vi "AlliGator Select FLI Channel Type.vi"(0 "Available Channel Names":string[](array[string]), 11 "error in (no error)":errorcluster) -> (1 "Dataset Channel":T1, 2 "Available Channel Names":string[](array[string]), 3 "Complementary Channel Name":string, 4 "Selected Channel Name":string, 6 "Channel Arithmetic":T2, 10 "G2 Channel Name (or single Gate Name)":string, 13 "Selected Channel Message":string, 14 "INT Channel Name (or empty)":string, 15 "error out":errorcluster)   [LabVIEW 2021, in "AlliGator Dual-Channel Datasets.lvlib"]
doc: "Used when loading a new dataset. If the selected channel name is compatible, use it, if not either open a dialog (dual-channel dataset) or use the default (single-channel dataset)."
uses:
  AlliGator Dual-Channel Datasets.lvlib
  AlliGator Gate Arithmetic.ctl
  AlliGator Dataset Channel.ctl
  AlliGator Settings List.ctl
  Variant/Variant to Data/Variant to [String].vi
  Variant/Variant to Data/Variant to U16.vi
  AlliGator Settings.lvlib
  Variant/Variant to Data/Variant to Data.lvlib
  AlliGator HDF5.lvlib
  AlliGator Files.lvlib
panel:
  out "Cancelled?":bool
  # "see the AlliGator License on the block diagram (Ctrl+E or Window:Show Block Diagram)"
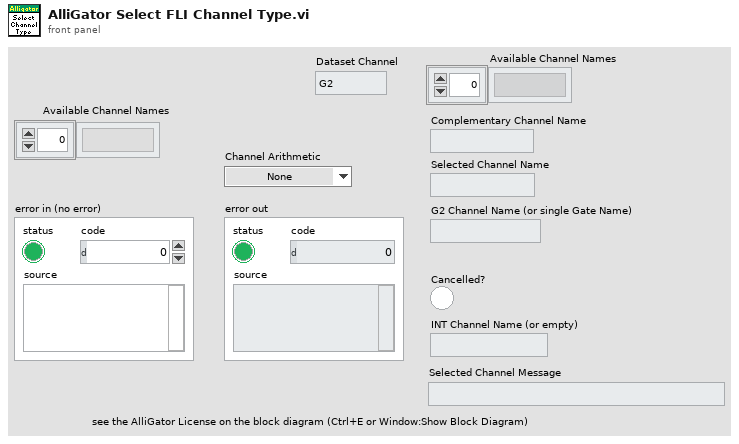
[diagram p1: front panel]
types:
  T1 = typedef "AlliGator Dual-Channel Datasets.lvlib/AlliGator Dataset Channel.ctl" = enum16{"G2", "INT"}
  T2 = typedef "AlliGator Settings.lvlib/AlliGator Gate Arithmetic.ctl" = enum16{"None", "INT-G2", "G2/INT*<INT>", "(1 - G2/INT)*<INT>"}
  T3 = typedef "AlliGator Settings.lvlib/AlliGator Settings List.ctl" = enum16{"GUI:Visible Settings Tab", "GUI:Last Run Version", "Source Image:Use Image Histogram for Contrast", "Source Image:Low Count Pixels Rejection Options", "Source Image:High Count Pixels Rejection Options", "Source Image:Use Image Brightness", "Source Image:Blend Overlay with Image Background", "Source Image:Use Fixed ROI Diameter", "Source Image:ROI Diameter", "Source Image:ROI Center Color", "Source Image:Peak Threshold", "Source Image:Intensity Threshold", "Source Image:Image Binning Options", "Source Image:Image Smoothing Options", "Source Image:Image Histogram Active", "Source Image:Invert Binary Mask", "Source Image:Hot Pixel Removal", "Source Image:Overlay Analyzed ROI Center", "Source Image:Auto-Adjust Contrast", "Source Image:Histogram Lower Percentile", "Source Image:Histogram Upper Percentile", "Source Image:Save Source Image", "Source Image:Scale Bar Options", "Source Image:Image Resolution (Pixel Size)", "Source Image:Flatfield Correction", "Source Image:Show Dead Left Columns Correction", "Source Image:Dead Left Columns Correction", "Source Image:Image Pre-Processing Operations Order", "Data Information:Gate Width", "Data Information:Nanotime Gate Separation", "Data Information:Macrotime Gate Separation", "Data Information:Gate Step", "Data Information:# Gates", "Data Information:Gate Image Exposure", "Data Information:Gate Image Integration", "Data Information:Gates to Skip", "Data Information:Gates to Keep", "Data Information:Define Gates to", "Data Information:Channel Name", "Data Information:Available Channel Names", "Data Information:Channel Arithmetic", "Data Information:Background File Subtraction", "Data Information:Background File", "Data Information:Background Scaling Factor", "Data Information:Background Pile-up Correction", "Data Information:Background Pixel Well Capacity", "Data Information:Laser Period", "Data Information:SYNC Period", "Data Information:Pile-up Correction", "Data Information:Pixel Well Capacity", "Data Information:Dataset Scaling Factor", "Fluorescence Decay_Decay Pre-Processing:Reverse Gates", "Fluorescence Decay_Decay Pre-Processing:Verbose Decay Pre-Processing", "Fluorescence Decay_Decay Pre-Processing:Use Decay Pre-Processing", "Fluorescence Decay_Decay Pre-Processing:Background Subtraction", "Fluorescence Decay_Decay Pre-Processing:Background Definition Range", "Fluorescence Decay_Decay Pre-Processing:Baseline Subtraction Method", "Fluorescence Decay_Decay Pre-Processing:Decay Pre-Processing Operations Order", "Fluorescence Decay_Decay Pre-Processing:Smoothing Parameter", "Fluorescence Decay_Decay Pre-Processing:Shift Decay", "Fluorescence Decay_Decay Pre-Processing:Decay Shift Parameters", "Fluorescence Decay_Decay Pre-Processing:Fold Decay", "Fluorescence Decay_Decay Pre-Processing:# Folds", "Fluorescence Decay_Decay Pre-Processing:1-Normalize Decay", "Fluorescence Decay_Decay Pre-Processing:[0-1]-Normalize Decay", "Fluorescence Decay_Decay Pre-Processing:Smoothen Decay", "Fluorescence Decay_Decay Pre-Processing:Extrapolate Decay", "Fluorescence Decay_Decay Pre-Processing:Use Periodicity", "Fluorescence Decay_Decay Pre-Processing:Use Cursors", "Fluorescence Decay_Decay Pre-Processing:Tail Fraction", "Fluorescence Decay_Decay Pre-Processing:Head Fraction", "Fluorescence Decay_Decay Pre-Processing:Additional Points", "Fluorescence Decay_Decay Pre-Processing:Straighten Decay", "Fluorescence Decay_Decay Pre-Processing:Constant Background", "Fluorescence Decay_Decay Pre-Processing:Pixel-Normalize Decay", "Fluorescence Decay_Advanced Analysis:Extract IRF instead of Decay", "Fluorescence Decay_Advanced Analysis:IRF Extraction Options", "Fluorescence Decay_Advanced Analysis:IRF Optimization Options", "Fluorescence Decay_Advanced Analysis:Square Pulse Options", "Fluorescence Decay_Advanced Analysis:IRF Order", "Fluorescence Decay_Advanced Analysis:IRF Time Constants", "Fluorescence Decay_Advanced Analysis:Wavelet Analysis Options", "Fluorescence Decay_Advanced Analysis:Average Lifetime Options", "Fluorescence Decay_Fit Options:Fit Options", "Fluorescence Decay_Fit Options:Use Legacy Fitting Approach", "Fluorescence Decay_Fit Options:Use Data Information Laser Period", "Fluorescence Decay_Fit Parameters:Displayed Fit Parameters", "Fluorescence Decay_Fit Parameters:Fit Parameter Constraints", "Fluorescence Decay_Fit Parameters:Export Tabulated Results", "Fluorescence Decay_Fit Parameters:MLE Baseline Offset Type", "Fluorescence Decay_Fit Parameters:MLE Baseline Offset", "Fluorescence Decay_Fit Parameters:Guess Parameter Names", "Fluorescence Decay_Fit Parameters:Guess Parameter Values", "Fluorescence Decay_Fit Parameters:Guess Parameters Options", "Fluorescence Decay_Styles:Show Last Decay Only", "Fluorescence Decay_Styles:Decay Graph Color Array", "Fluorescence Decay:Decay Graph Active", "Fluorescence Decay Statistics:Min Peak Value", "Fluorescence Decay Statistics:Reject Low Decay Peak Pixels", "Fluorescence Decay Statistics:Reject High Decay Peak Pixels", "Fluorescence Decay Statistics:Max Peak Value", "Time Traces:Use File Timestamp", "Time Traces:Time Step", "Time Traces:Use Intensity Correction File", "Time Traces:Intensity Correction File", "Phasor Plot:Phasor Plot Smoothing Options", "Phasor Plot:Phasor Plot Size", "Phasor Plot:Phasor Plot Graphics Options", "Phasor Plot:Cumulative Phasor Plot", "Phasor Plot:Use Phasor Brightness", "Phasor Plot:Blend Overlay with Phasor Background", "Phasor Plot:Save Phasor Plot", "Phasor Plot:Show References", "Phasor Plot:Phasor Ratio Decay Range", "Phasor Plot:Exponential Fading", "Phasor Plot:Phasor Ratio Reference Colors", "Phasor Plot:Reference Radius", "Phasor Plot:Show Color Map Vertices", "Phasor Plot:Phasor Plot Active", "Phasor Plot:Phasor Ratio Color Map Type", "Phasor Plot:Phasor Ratio Color Map", "Phasor Plot:Phasor Ratio Display Range", "Phasor Plot:Selected Image ROI(s)", "Phasor Plot:All Image ROIs", "Phasor Plot:Selected Phasor Plot ROI(s)", "Phasor Plot:All Phasor Plot ROIs", "Phasor Plot:Phasor Ratio Color-Coded Quantity", "Phasor Plot:Store Phasor Harmonics", "Phasor Plot:Draw Reference Segment", "Phasor Plot:User-Defined Quantity", "Phasor Graph:Phasor Frequency", "Phasor Graph:Phasor Ratio Type", "Phasor Graph:Pixel-level Phasor Computation", "Phasor Graph:Save Phasor Graph", "Phasor Graph:Phasor Graph Active", "Phasor Graph:Phasor SDV Options", "Phasor Calibration:Use Backup Calibration if needed", "Phasor Graph:Define Shortest Lifetime as", "Phasor Calibration:Backup Calibration Type", "Phasor Calibration:Calibration Type", "Phasor Calibration:Calibration Lifetime", "Phasor Calibration:Calibration Map Algorithm", "Single-Exponential Phasor Locus (SEPL):Gate Parameters", "Single-Exponential Phasor Locus (SEPL):User-defined Gate", "Single-Exponential Phasor Locus (SEPL):User-defined IRF", "Single-Exponential Phasor Locus (SEPL):Phasor Parameters", "Single-Exponential Phasor Locus (SEPL):Decay & IRF Parameters", "Single-Exponential Phasor Locus (SEPL):Display Parameters", "Lifetime Analysis:Decay Analysis Parameters", "Lifetime Analysis:Lifetime Map Active", "Plugins:Python Settings", "Miscellaneous:Verbose Mode", "Miscellaneous:Beep after Script", "Miscellaneous:Saved Image File Format", "Miscellaneous:Exported Gate Image Settings", "Miscellaneous:Include Loading in Timing", "Miscellaneous:Verbose Settings Mode", "Miscellaneous:Histogram Options", "Miscellaneous:Beep on Error", "Miscellaneous:# Logical Processors Used", "Miscellaneous:ROI Description Max Characters", "Miscellaneous:Verbose Error Mode", "Miscellaneous:Transparent Mask Color"}
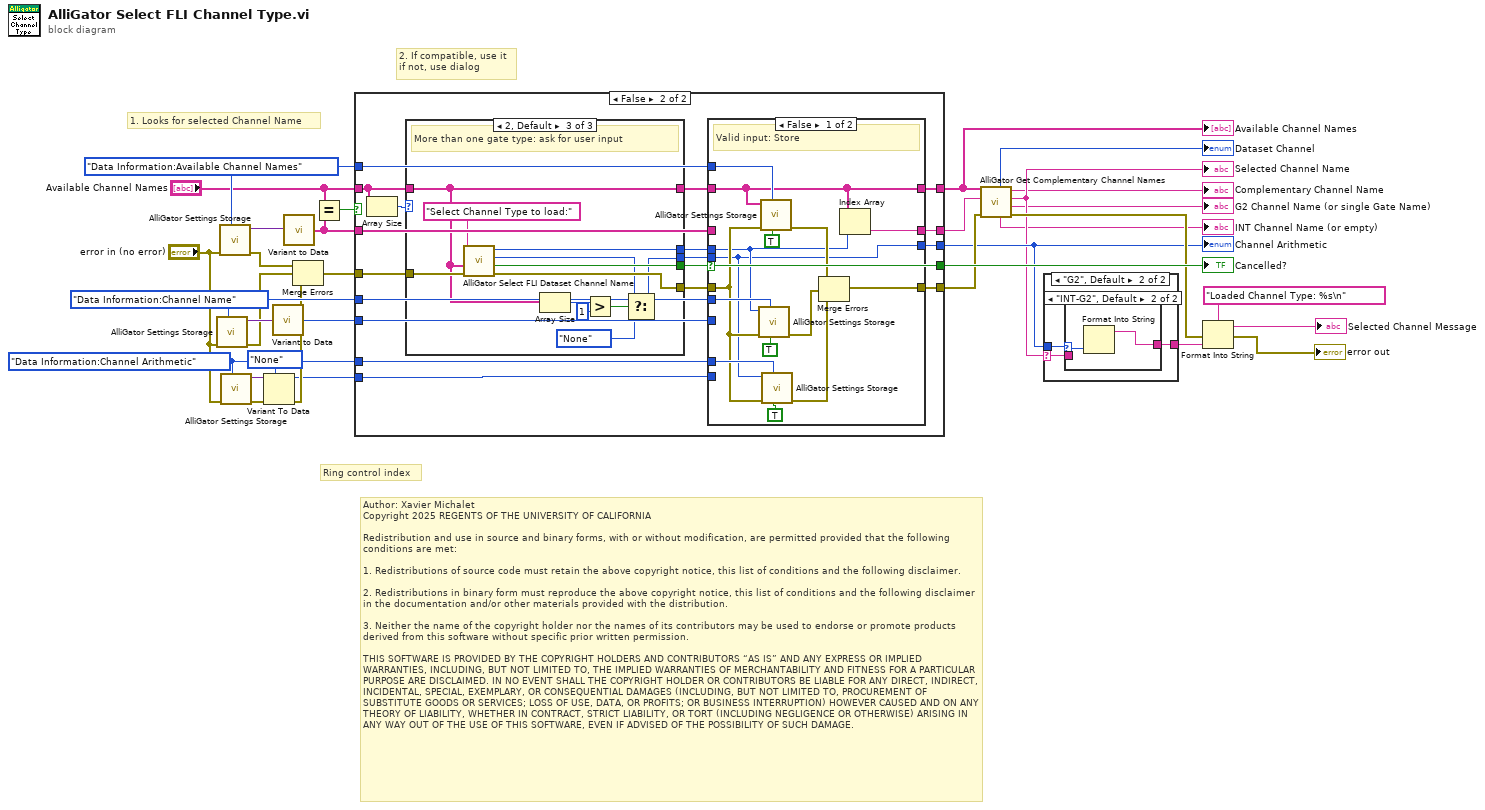
[diagram p0: block diagram]
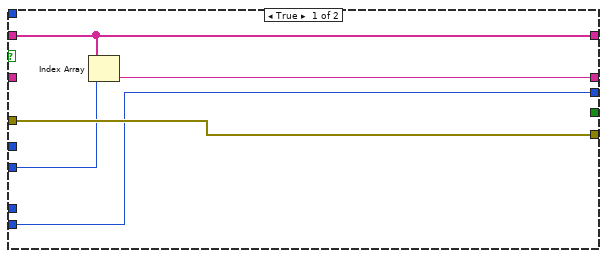
[diagram p4: hidden frame]
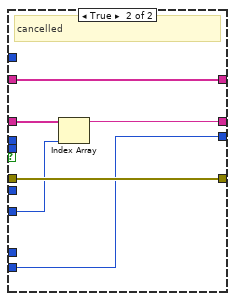
[diagram p5: hidden frame]
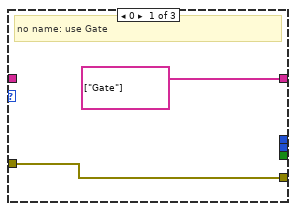
[diagram p6: hidden frame]
diagram:
  w22 = AlliGator_Settings_List."Data Information:Channel Arithmetic" ("AlliGator Settings List")
  w25 = AlliGator_Settings_List."Data Information:Channel Name" ("AlliGator Settings List")
  w26 = AlliGator_Settings_List."Data Information:Available Channel Names" ("AlliGator Settings List")
  # "Author: Xavier Michalet\nCopyright 2025 REGENTS OF THE UNIVERSITY OF CALIFORNIA\n\nRedistribution and use in source and binary forms, with or without modification, are permitted provided that the following conditions are met:\n\n1. Redistributions of source code must retain the above copyright notice, this list of conditions and the following disclaimer.\n\n2. Redistributions in binary form must reproduce the above copyright notice, this list of conditions and the following disclaimer in the documentation and/or other materials provided with the distribution.\n\n3. Neither the name of the copyright holder nor the names of its contributors may be used to endorse or promote products derived from this software without specific prior written permission.\n\nTHIS SOFTWARE IS PROVIDED BY THE COPYRIGHT HOLDERS AND CONTRIBUTORS “AS IS” AND ANY EXPRESS OR IMPLIED WARRANTIES, INCLUDING, BUT NOT LIMITED TO, THE IMPLIED WARRANTIES OF MERCHANTABILITY AND FITNESS FOR A PARTICULAR PURPOSE ARE DISCLAIMED. IN NO EVENT SHALL THE COPYRIGHT HOLDER OR CONTRIBUTORS BE LIABLE FOR ANY DIRECT, INDIRECT, INCIDENTAL, SPECIAL, EXEMPLARY, OR CONSEQUENTIAL DAMAGES (INCLUDING, BUT NOT LIMITED TO, PROCUREMENT OF SUBSTITUTE GOODS OR SERVICES; LOSS OF USE, DATA, OR PROFITS; OR BUSINESS INTERRUPTION) HOWEVER CAUSED AND ON ANY THEORY OF LIABILITY, WHETHER IN CONTRACT, STRICT LIABILITY, OR TORT (INCLUDING NEGLIGENCE OR OTHERWISE) ARISING IN ANY WAY OUT OF THE USE OF THIS SOFTWARE, EVEN IF ADVISED OF THE POSSIBILITY OF SUCH DAMAGE."
  # "Ring control index"
  # "2. If compatible, use it\nif not, use dialog"
  # "1. Looks for selected Channel Name"
  n1 = call "AlliGator Settings Storage.vi"("AlliGator Settings List"=w25, "Error In"="error in (no error)") -> ("Error Out"=w30:errorcluster, "Variant Data out"=w33:variant)  [unwired: 8 in]
  n2 = call "AlliGator Settings Storage.vi"("AlliGator Settings List"=w26, "Error In"="error in (no error)") -> ("Error Out"=w31:errorcluster, "Variant Data out"=w32:variant)  [unwired: 8 in]
  n3 = call "AlliGator Settings Storage.vi"("AlliGator Settings List"=w22, "Error In"="error in (no error)") -> ("Error Out"=w10:errorcluster, "Variant Data out"=w11:variant)  [unwired: 8 in]
  n4 = Variant To Data(error in=w10, type=AlliGator_Gate_Arithmetic."None" ("Gate Arithmetic"), Variant=w11) -> (data=w7:T2, error out=w9:errorcluster)
  n5 = call-poly "Variant to Data.vi"("Variant"=w33) -> ("U16 Value"=w28:u16)  [unwired: 8 in]
  n6 = call-poly "Variant to Data.vi"("Variant"=w32) -> ("String Array"=w24:string[])  [unwired: 8 in]
  n7 = Merge Errors(w31, w30, w9) -> (w29:errorcluster)
  n8 = Equal?(x="Available Channel Names", y=w24) -> (x = y?=w27:bool)
  n9 = case shown="False" w27 {
    tunnel: [w36 w49] -> w15
    tunnel: w29 -> [w38 w56]
    tunnel: [w38 w50] -> w14
    tunnel: "Available Channel Names" -> [w34 w46]
    tunnel: [_ w54] -> w18
    tunnel: w28 -> [w37 w47]
    tunnel: w26 -> [_ w53]
    tunnel: w25 -> [_ w51]
    tunnel: w24 -> [_ w48]
    tunnel: w7 -> [w35 w41]
    tunnel: [w35 w42] -> w6
    tunnel: w22 -> [_ w40]
    tunnel: [w34 w39] -> w16
    frame True {
      n10 = Index Array(array=w34, index=w37) -> (element=w36:string)
    }
    frame False {
      n11 = Array Size(array=w46) -> (size(s)=w45:i32)
      n12 = case shown="2, Default" w45 {
        tunnel: w56 -> [w78 w80 w93]
        tunnel: [w78 w80 w91] -> w55
        tunnel: [_ _ w90] -> w54
        tunnel: [_ _ w89] -> w52
        tunnel: w46 -> [_ w81 w84]
        tunnel: [string[] ["Gate"] ("Available Gate Names") w81 w84] -> w44
        tunnel: [_ _ w82] -> w43
        frame 0 {
          # "no name: use Gate"
        }
        frame 1 {
          # "single gate type: no need for user rinput"
        }
        frame 2, Default {
          # "More than one gate type: ask for user input"
          n13 = call "AlliGator Select FLI Dataset Channel Name.vi"("Error In"=w93, "Channel Names"=w84, "Input Message"="Select Channel Type to load:") -> ("Error Out"=w91:errorcluster, "Cancelled?"=w90:bool, "Channel Arithmetic"=w83:T2, "Selected Channel"=w89:u16)  [unwired: 5 in]
          n14 = Array Size(array=w84) -> (size(s)=w88:i32)
          n15 = Greater?(x=w88, y=1) -> (0:w86:bool)
          n16 = Select(t=w83, s=w86, f=AlliGator_Gate_Arithmetic."None") -> (s? t:f=w82:T2)
        }
      }
      n17 = case shown="False" w54 {
        tunnel: w55 -> [w62 w77]
        tunnel: w53 -> [w69 _]
        tunnel: w44 -> [w59 w72]
        tunnel: w52 -> [w58 _]
        tunnel: w51 -> [w66 _]
        tunnel: [w71 w77] -> w50
        tunnel: [w70 w74] -> w49
        tunnel: w48 -> [_ w76]
        tunnel: w47 -> [_ w75]
        tunnel: w43 -> [w57 _]
        tunnel: [w57 w73] -> w42
        tunnel: w41 -> [_ w73]
        tunnel: w40 -> [w63 _]
        tunnel: [w59 w72] -> w39
        frame False {
          # "Valid input: Store"
          n18 = call "AlliGator Settings Storage.vi"("Get(F)/Set"=TRUE, "AlliGator Settings List"=w66, "Error In"=w62, "Variant Data in"=w58) -> ("Error Out"=w65:errorcluster)  [unwired: 6 in, 1 out]
          n19 = call "AlliGator Settings Storage.vi"("Get(F)/Set"=TRUE, "AlliGator Settings List"=w69, "Error In"=w62, "Variant Data in"=w59) -> ("Error Out"=w68:errorcluster)  [unwired: 6 in, 1 out]
          n20 = call "AlliGator Settings Storage.vi"("Get(F)/Set"=TRUE, "AlliGator Settings List"=w63, "Error In"=w62, "Variant Data in"=w57) -> ("Error Out"=w61:errorcluster)  [unwired: 6 in, 1 out]
          n21 = Merge Errors(w68, w65, w61) -> (w71:errorcluster)
          n22 = Index Array(array=w59, index=w58) -> (element=w70:string)
        }
        frame True {
          # "cancelled"
          n23 = Index Array(array=w76, index=w75) -> (element=w74:string)
        }
      }
    }
  }
  "Cancelled?" <- w18
  "Channel Arithmetic" <- w6
  "Available Channel Names" <- w16
  n24 = call "AlliGator Get Complementary Channel Names.vi"("Error In"=w14, "Selected Channel Name"=w15, "Available Channel Names"=w16) -> ("Error Out"=w13:errorcluster, "G2 Channel Name (or single Gate Name)"=→"G2 Channel Name (or single Gate Name)":string, "Selected Channel Name (dup)"=w5:string, "Complementary Channel Name (or empty)"=→"Complementary Channel Name":string, "INT Channel Name (or empty)"=→"INT Channel Name (or empty)":string, "Dataset Channel"=→"Dataset Channel":T1)  [unwired: 3 in]
  "Selected Channel Name" <- w5
  n25 = case shown="\"G2\", Default" w5 {
    selector: w5 -> [w94 w95]
    tunnel: [w94 w96] -> w19
    tunnel: w6 -> [_ w97]
    frame "Gate" {
    }
    frame "G2", Default {
      n26 = case shown="\"INT-G2\", Default" w97 {
        selector: w97 -> [_ w100]
        tunnel: [w98 w99] -> w96
        tunnel: w95 -> [w98 _]
        frame "None" {
        }
        frame "INT-G2", Default {
          n27 = Format Into String(w100) -> (resulting string=w99:string)  [unwired: 3 in, 1 out]
        }
      }
    }
  }
  n28 = Format Into String(format string="Loaded Channel Type: %s\n", error in=w13, w19) -> (resulting string=→"Selected Channel Message":string, error out=→"error out":errorcluster)  [unwired: 1 in]
